vi "SDCP SMF Rx Logger - FGV.vi"(0 "Commands":T2, 1 "error in (no error)":errorcluster) -> (2 "Instantaeneous logged data":T1[](array[typedef]), 3 "Complete logged data":T1[](array[typedef]), 4 "error out":errorcluster)   [LabVIEW 2020]
uses:
  SDCP SMF Rx Logger - FGV - Commands.vi
  Typedefs/SDCP SMF logger - SMF with timestamp.ctl
  Typedefs/SDCP SMF Rx Logger - Notifier FGV - Notifier names.ctl
  Typedefs/SDCP SMF Rx Logger - Notifier FGV - Commands.ctl
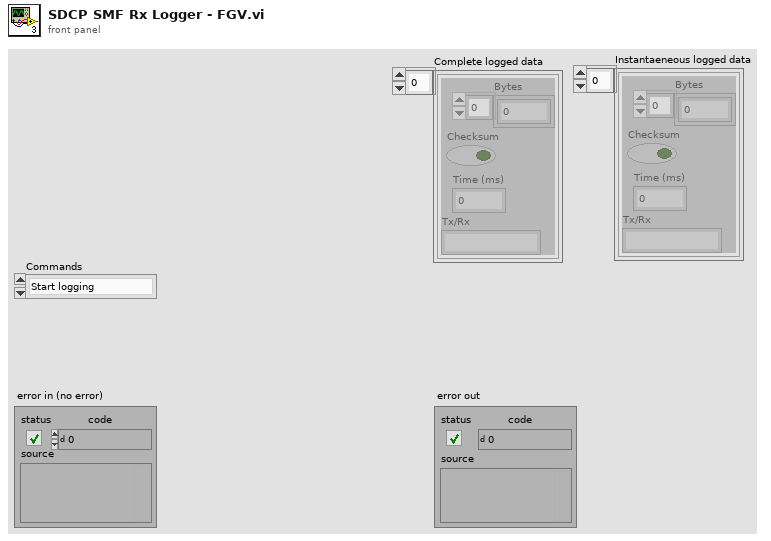
[diagram p1: front panel]
types:
  T1 = typedef "SDCP SMF logger - SMF with timestamp.ctl" = cluster{"Bytes":u8[], "Checksum":bool, "Time (ms)":u32, "Tx/Rx":string}
  T2 = typedef "SDCP SMF Rx Logger - FGV - Commands.vi" = enum16{"Start logging", "Pause logging", "Get log data", "Reset log", "Stop logging"}
  T3 = typedef "SDCP SMF Rx Logger - Notifier FGV - Commands.ctl" = enum16{"Initialize", "Read", "Write", "Deinitialize"}
  T4 = typedef "SDCP SMF Rx Logger - Notifier FGV - Notifier names.ctl" = enum16{"Logged data", "Pause logging", "Get log", "Reset log", "Sample counter", "Logged data buffer", "Stop logging"}
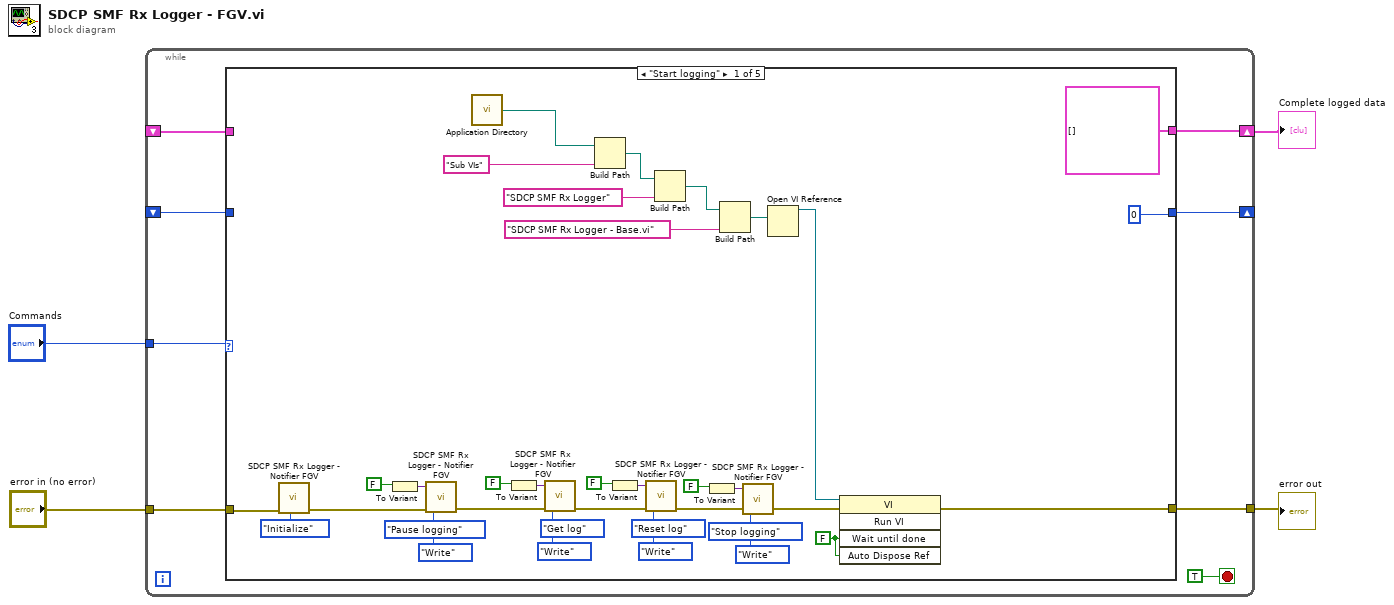
[diagram p0: block diagram]
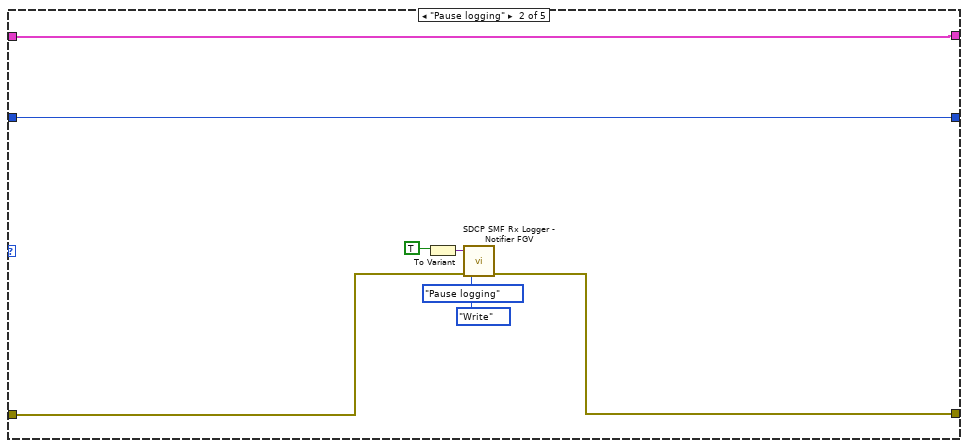
[diagram p2: hidden frame]
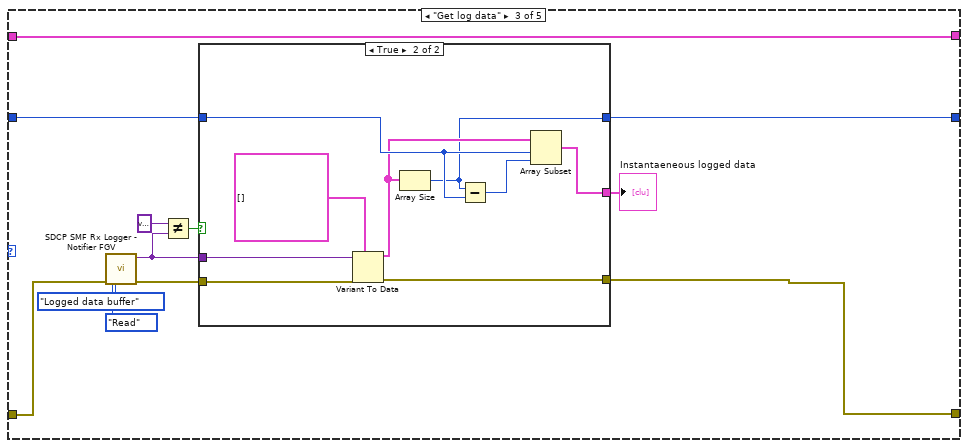
[diagram p3: hidden frame]
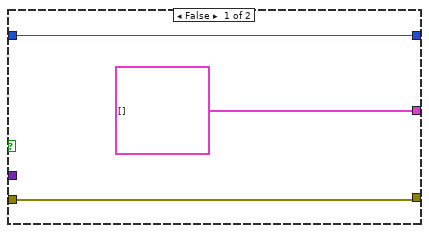
[diagram p4: hidden frame]
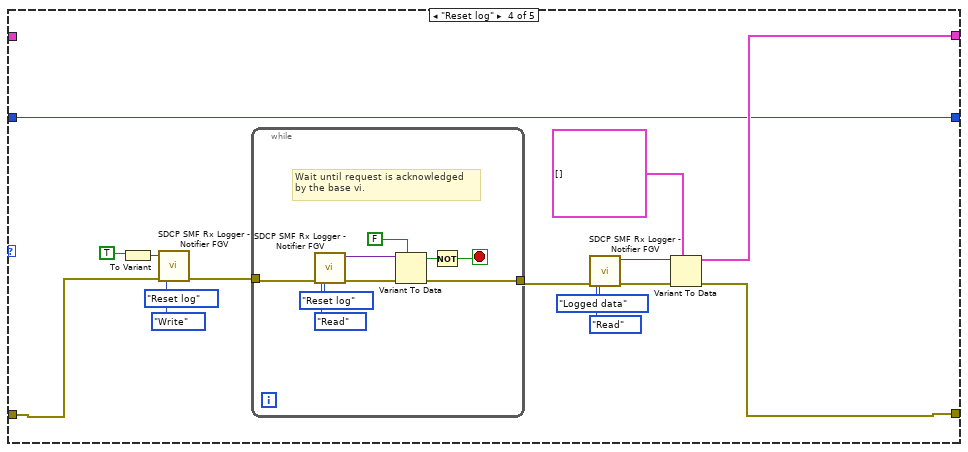
[diagram p5: hidden frame]
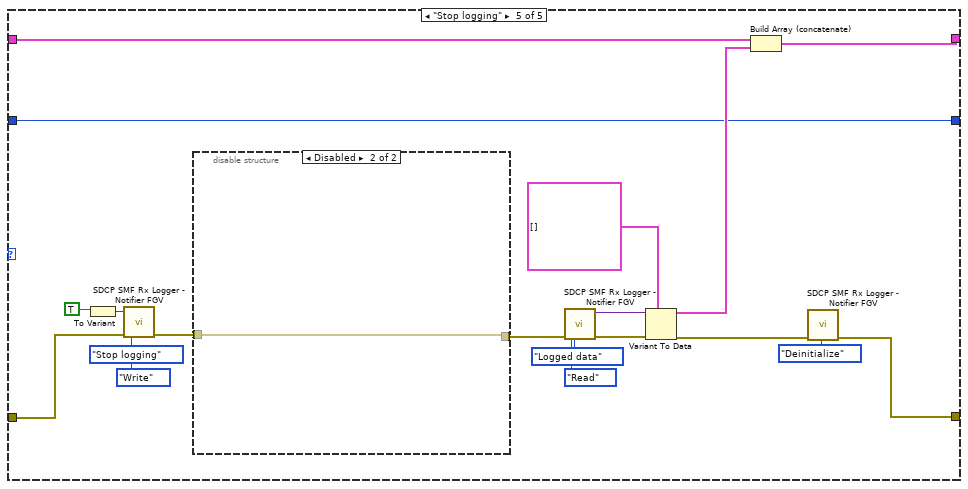
[diagram p6: hidden frame]
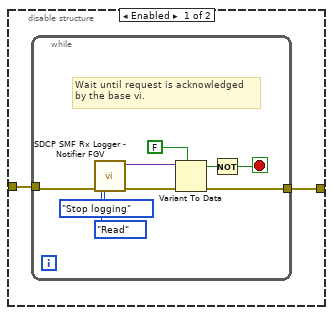
[diagram p7: hidden frame]
diagram:
  n1 = while {
    tunnel: "error in (no error)" -> [w10]
    tunnel: "Commands" -> [w11]
    tunnel: [w9] -> w2
    shift-right: [w7] -> w1
    shift-left: _ -> [w8]
    shift-right: [w5] -> _
    shift-left: _ -> [w6]
    stop <- TRUE stop-if-true
    n2 = case shown="\"Start logging\"" w11 {
      tunnel: w10 -> [w47 w51 w63 w83 w117]
      tunnel: [w18 w50 w59 w82 w105] -> w9
      tunnel: w8 -> [_ w49 w64 _ w110]
      tunnel: [T1[] [] w49 w64 w81 w108] -> w7
      tunnel: w6 -> [_ w48 w58 w80 w104]
      tunnel: [0 w48 w57 w80 w104] -> w5
      frame "Start logging" {
        w19 = FALSE ("Wait Until Done")
        n3 = call "SDCP SMF Rx Logger - Notifier FGV.vi"("error in (no error)"=w47, "Command"=SDCP_SMF_Rx_Logger_-_Notifier_FGV_-_Commands."Initialize") -> ("error out"=w45:errorcluster)  [unwired: 4 in, 1 out]
        n4 = To Variant(anything=FALSE) -> (Variant=w42:variant)
        n5 = call "SDCP SMF Rx Logger - Notifier FGV.vi"("error in (no error)"=w45, "Command"=SDCP_SMF_Rx_Logger_-_Notifier_FGV_-_Commands."Write", "Notifier name"=SDCP_SMF_Rx_Logger_-_Notifier_FGV_-_Notifier_names."Pause logging", "Notifier value in"=w42) -> ("error out"=w36:errorcluster)  [unwired: 2 in, 1 out]
        n6 = call <vilib>:"Application Directory.vi"() -> ("Application Directory"=w14:path)
        n7 = To Variant(anything=FALSE) -> (Variant=w38:variant)
        n8 = call "SDCP SMF Rx Logger - Notifier FGV.vi"("error in (no error)"=w36, "Command"=SDCP_SMF_Rx_Logger_-_Notifier_FGV_-_Commands."Write", "Notifier name"=SDCP_SMF_Rx_Logger_-_Notifier_FGV_-_Notifier_names."Get log", "Notifier value in"=w38) -> ("error out"=w31:errorcluster)  [unwired: 2 in, 1 out]
        n9 = Build Path(base path=w14, name or relative path="Sub VIs") -> (appended path=w15:path)
        n10 = To Variant(anything=FALSE) -> (Variant=w33:variant)
        n11 = call "SDCP SMF Rx Logger - Notifier FGV.vi"("error in (no error)"=w31, "Command"=SDCP_SMF_Rx_Logger_-_Notifier_FGV_-_Commands."Write", "Notifier name"=SDCP_SMF_Rx_Logger_-_Notifier_FGV_-_Notifier_names."Reset log", "Notifier value in"=w33) -> ("error out"=w26:errorcluster)  [unwired: 2 in, 1 out]
        n12 = Build Path(base path=w15, name or relative path="SDCP SMF Rx Logger") -> (appended path=w24:path)
        n13 = To Variant(anything=FALSE) -> (Variant=w28:variant)
        n14 = Build Path(base path=w24, name or relative path="SDCP SMF Rx Logger - Base.vi") -> (appended path=w22:path)
        n15 = call "SDCP SMF Rx Logger - Notifier FGV.vi"("error in (no error)"=w26, "Command"=SDCP_SMF_Rx_Logger_-_Notifier_FGV_-_Commands."Write", "Notifier name"=SDCP_SMF_Rx_Logger_-_Notifier_FGV_-_Notifier_names."Stop logging", "Notifier value in"=w28) -> ("error out"=w21:errorcluster)  [unwired: 2 in, 1 out]
        n16 = Open VI Reference(vi path=w22) -> (vi reference=w20:refnum<vi>)  [unwired: 5 in, 1 out]
        n17 = invoke class="VI" method="Run VI"(reference=w20, error in=w21, "Wait until done"=w19, "Auto Dispose Ref"=w19) -> (error out=w18:errorcluster)  [unwired: 1 in, 4 out]
      }
      frame "Pause logging" {
        n18 = To Variant(anything=TRUE) -> (Variant=w53:variant)
        n19 = call "SDCP SMF Rx Logger - Notifier FGV.vi"("error in (no error)"=w51, "Command"=SDCP_SMF_Rx_Logger_-_Notifier_FGV_-_Commands."Write", "Notifier name"=SDCP_SMF_Rx_Logger_-_Notifier_FGV_-_Notifier_names."Pause logging", "Notifier value in"=w53) -> ("error out"=w50:errorcluster)  [unwired: 2 in, 1 out]
      }
      frame "Get log data" {
        n20 = call "SDCP SMF Rx Logger - Notifier FGV.vi"("error in (no error)"=w63, "Command"=SDCP_SMF_Rx_Logger_-_Notifier_FGV_-_Commands."Read", "Notifier name"=SDCP_SMF_Rx_Logger_-_Notifier_FGV_-_Notifier_names."Logged data buffer") -> ("error out"=w65:errorcluster, "Notifier value out"=w61:variant)  [unwired: 3 in]
        n21 = Not Equal?(x=variant, y=w61) -> (x != y?=w62:bool)
        n22 = case shown="True" w62 {
          tunnel: w65 -> [w70 w79]
          tunnel: w61 -> [_ w78]
          tunnel: [w70 w77] -> w59
          tunnel: [T1[] [] w72] -> w56
          tunnel: w58 -> [w68 w75]
          tunnel: [w68 w71] -> w57
          frame False {
          }
          frame True {
            n23 = Variant To Data(error in=w79, type=T1[] [], Variant=w78) -> (data=w73:T1[], error out=w77:errorcluster)
            n24 = Array Size(array=w73) -> (size(s)=w71:i32)
            n25 = Subtract(x=w71, y=w75) -> (x-y=w74:i32)
            n26 = Array Subset(array=w73, index=w75, length=w74) -> (w72:T1[])
          }
        }
        "Instantaeneous logged data" <- w56
      }
      frame "Reset log" {
        n27 = To Variant(anything=TRUE) -> (Variant=w92:variant)
        n28 = call "SDCP SMF Rx Logger - Notifier FGV.vi"("error in (no error)"=w83, "Command"=SDCP_SMF_Rx_Logger_-_Notifier_FGV_-_Commands."Write", "Notifier name"=SDCP_SMF_Rx_Logger_-_Notifier_FGV_-_Notifier_names."Reset log", "Notifier value in"=w92) -> ("error out"=w90:errorcluster)  [unwired: 2 in, 1 out]
        n29 = while {
          tunnel: w90 -> [w103]
          tunnel: [w95] -> w85
          stop <- w96 stop-if-true
          # "Wait until request is acknowledged\nby the base vi."
          n30 = call "SDCP SMF Rx Logger - Notifier FGV.vi"("error in (no error)"=w103, "Command"=SDCP_SMF_Rx_Logger_-_Notifier_FGV_-_Commands."Read", "Notifier name"=SDCP_SMF_Rx_Logger_-_Notifier_FGV_-_Notifier_names."Reset log") -> ("error out"=w100:errorcluster, "Notifier value out"=w98:variant)  [unwired: 3 in]
          n31 = Variant To Data(error in=w100, type=FALSE, Variant=w98) -> (data=w97:bool, error out=w95:errorcluster)
          n32 = Not(x=w97) -> (.not. x?=w96:bool)
        }
        n33 = call "SDCP SMF Rx Logger - Notifier FGV.vi"("error in (no error)"=w85, "Command"=SDCP_SMF_Rx_Logger_-_Notifier_FGV_-_Commands."Read", "Notifier name"=SDCP_SMF_Rx_Logger_-_Notifier_FGV_-_Notifier_names."Logged data") -> ("error out"=w87:errorcluster, "Notifier value out"=w86:variant)  [unwired: 3 in]
        n34 = Variant To Data(error in=w87, type=T1[] [], Variant=w86) -> (data=w81:T1[], error out=w82:errorcluster)
      }
      frame "Stop logging" {
        n35 = To Variant(anything=TRUE) -> (Variant=w120:variant)
        n36 = call "SDCP SMF Rx Logger - Notifier FGV.vi"("error in (no error)"=w117, "Command"=SDCP_SMF_Rx_Logger_-_Notifier_FGV_-_Commands."Write", "Notifier name"=SDCP_SMF_Rx_Logger_-_Notifier_FGV_-_Notifier_names."Stop logging", "Notifier value in"=w120) -> ("error out"=w118:errorcluster)  [unwired: 2 in, 1 out]
        n37 = disable-structure shown="Disabled" {
          disable-tunnel: w118 -> [w124 w134]
          disable-tunnel: [w123 w134] -> w111
          frame Enabled {
            n38 = while {
              tunnel: w124 -> [w133]
              tunnel: [w125] -> w123
              stop <- w126 stop-if-true
              # "Wait until request is acknowledged\nby the base vi."
              n39 = call "SDCP SMF Rx Logger - Notifier FGV.vi"("error in (no error)"=w133, "Command"=SDCP_SMF_Rx_Logger_-_Notifier_FGV_-_Commands."Read", "Notifier name"=SDCP_SMF_Rx_Logger_-_Notifier_FGV_-_Notifier_names."Stop logging") -> ("error out"=w130:errorcluster, "Notifier value out"=w128:variant)  [unwired: 3 in]
              n40 = Variant To Data(error in=w130, type=FALSE, Variant=w128) -> (data=w127:bool, error out=w125:errorcluster)
              n41 = Not(x=w127) -> (.not. x?=w126:bool)
            }
          }
          frame Disabled {
          }
        }
        n42 = call "SDCP SMF Rx Logger - Notifier FGV.vi"("error in (no error)"=w111, "Command"=SDCP_SMF_Rx_Logger_-_Notifier_FGV_-_Commands."Read", "Notifier name"=SDCP_SMF_Rx_Logger_-_Notifier_FGV_-_Notifier_names."Logged data") -> ("error out"=w114:errorcluster, "Notifier value out"=w113:variant)  [unwired: 3 in]
        n43 = Variant To Data(error in=w114, type=T1[] [], Variant=w113) -> (data=w109:T1[], error out=w107:errorcluster)
        n44 = Build Array (concatenate)(w110, w109) -> (w108:T1[])
        n45 = call "SDCP SMF Rx Logger - Notifier FGV.vi"("error in (no error)"=w107, "Command"=SDCP_SMF_Rx_Logger_-_Notifier_FGV_-_Commands."Deinitialize") -> ("error out"=w105:errorcluster)  [unwired: 4 in, 1 out]
      }
    }
  }
  "error out" <- w2
  "Complete logged data" <- w1
